vi "Testing HW control panel.vi"() -> ()   [LabVIEW 2009]
uses:
  <vilib>/rvi/interface/nirviOpenFPGA/nirviOpenFPGA.xnode
  <vilib>/userDefined/High Color/nirio_resource_hc.ctl
  <vilib>/rvi/interface/nirviCloseFPGA/nirviCloseFPGA.xnode
  FPGA Bitfiles/Q_IGVC_2010.lvproj_FPGA Target_HW Control Panel F~C3.lvbitx
  <vilib>/rvi/interface/nirviReadWriteControl/nirviReadWriteControl.xnode
  NiRioSrv.dll
  <vilib>/Utility/error.llb/Error Cluster From Error Code.vi
  <vilib>/rvi/errors/niLvFpgaWhatHappensToTopLevelVI.ctl
  <vilib>/rvi/interface/common/niFpgaNodeNameForErrorReporting.ctl
  <vilib>/rvi/errors/niLvFpgaAdjustHostInterfaceError.vi
  <vilib>/FPGAPlugInAG/cRIO-9113/nirviIntfOpen_cRIO-9113.vi
  <vilib>/RVI Host/nirviSupport.llb/nirviErrorClusterFromErrorCode.vi
  FPGA/Control Panel/Hardware Control Panel States.ctl
  <vilib>/FPGAPlugInAG/cRIO-9113/nirviIntfClose_cRIO-9113.vi
panel:
  in  "HB LED Multiple":u32=500
  in  "Safety LED Multiple":u32=500
  in  "Init LED Multiple":u32=500
  out "Go Button":bool
  out "Safety Switch":bool
  out "Init Switch":bool
  out "Current Control Panel State":T1
  in  "Init Complete in":bool
  in  "Safety Disabled":bool
  out "Init Complete":bool
  out "Init LED ON/OFF/BLINK":u8
  in  "stop":bool
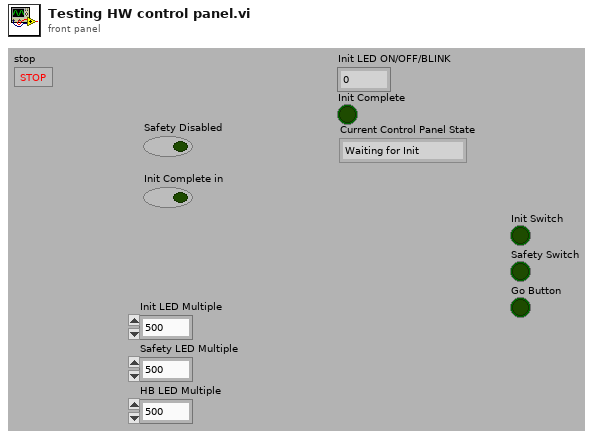
[diagram p1: front panel]
types:
  T1 = typedef "Hardware Control Panel States.ctl" = enum16{"Waiting for Init", "Init", "Waiting for Safety", "Safety", "Waiting for GO", "GO"}
  T2 = typedef "nirio_resource_hc.ctl" = tag
  T3 = typedef "niFpgaNodeNameForErrorReporting.ctl" = enum16{"Open FPGA VI Reference", "Read/Write Control", "Invoke Method: Abort", "Invoke Method: Acknowledge IRQ", "Invoke Method: Download", "Invoke Method: FIFO.Configure", "Invoke Method: FIFO.Read", "Invoke Method: FIFO.Start", "Invoke Method: FIFO.Stop", "Invoke Method: FIFO.Write", "Invoke Method: Reset", "Invoke Method: Run", "Invoke Method: Wait on IRQ", "Close FPGA VI Reference"}
  T4 = typedef "niLvFpgaWhatHappensToTopLevelVI.ctl" = enum16{"top level VI scripted behind XNode", "top level VI inlined behind XNode"}
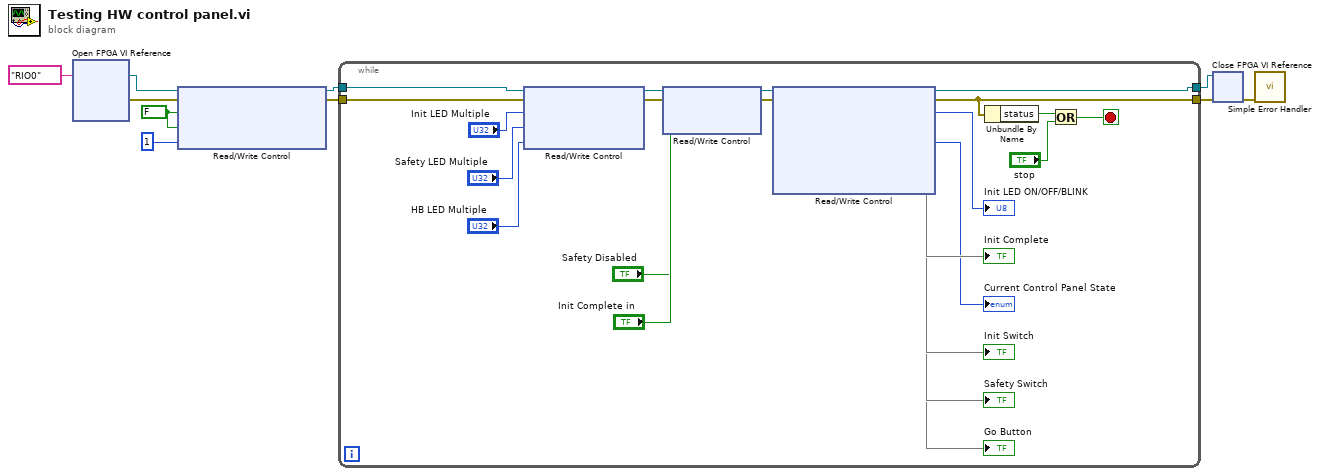
[diagram p0: block diagram]
diagram:
  w3 = FALSE ("Safety Disabled")
  n1 = xnode "Open FPGA VI Reference"("resource name"=T2 "RIO0") -> ("FPGA VI Reference Out"=w7:refnum<k20>, "error out"=w6:errorcluster)  [unwired: 1 in]
  n2 = xnode "Read/Write Control"("FPGA VI Reference In"=w7, "error in"=w6, "Safety Disabled"=w3, "Init Complete"=w3, "LED Control Loop Period"=u8 1) -> ("FPGA VI Reference Out"=w5:refnum<k20>, "error out"=w4:errorcluster)
  n3 = while {
    tunnel: [w31] -> w10
    tunnel: w5 -> [w17]
    tunnel: w4 -> [w16]
    tunnel: [w22] -> w9
    stop <- w23 stop-if-true
    n4 = xnode "Read/Write Control"("FPGA VI Reference In"=w17, "error in"=w16, "Init LED Multiple"="Init LED Multiple", "Safety LED Multiple"="Safety LED Multiple", "HB LED Multiple"="HB LED Multiple") -> ("FPGA VI Reference Out"=w14:refnum<k20>, "error out"=w15:errorcluster)
    n5 = xnode "Read/Write Control"("FPGA VI Reference In"=w14, "error in"=w15, "Safety Disabled"="Safety Disabled", "Init Complete"="Init Complete in") -> ("FPGA VI Reference Out"=w25:refnum<k20>, "error out"=w26:errorcluster)
    n6 = xnode "Read/Write Control"("FPGA VI Reference In"=w25, "error in"=w26) -> ("FPGA VI Reference Out"=w31:refnum<k20>, "error out"=w22:errorcluster, "Init LED ON/OFF/BLINK"=→"Init LED ON/OFF/BLINK":u8, "Init Complete"=→"Init Complete", "Current Control Panel State"=→"Current Control Panel State":T1, "Init Switch"=→"Init Switch", "Safety Switch"=→"Safety Switch", "Go Button"=→"Go Button")
    n7 = Unbundle By Name(w22) -> ("status"=w21:bool)
    n8 = Or(x=w21, y="stop") -> (x .or. y?=w23:bool)
  }
  n9 = xnode "Close FPGA VI Reference"("FPGA VI Reference In"=w10, "error in"=w9) -> ("error out"=w1:errorcluster)
  n10 = call <vilib>:"Simple Error Handler.vi"("error in (no error)"=w1) -> ()  [unwired: 4 in, 5 out]
